vi "Start Stop Integration.vi"(0 "VISA resource name":refnum<visa-resource-name>, 5 "Start/Stop (F: Stop)":bool, 11 "error in (no error)":errorcluster) -> (4 "VISA resource name out":refnum<visa-resource-name>, 15 "error out":errorcluster)   [LabVIEW 2011, in "Yokogawa WT200 Series.lvlib"]
doc: "This VI sends the Integrate start/stop command to the WT200 Series."
uses:
  G:/Engineering/Retail/LabV/instr.lib/Yokogawa WT200 Series/Yokogawa WT200 Series.lvlib
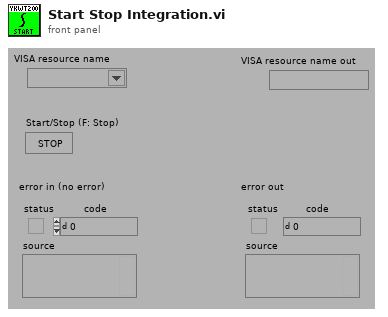
[diagram p1: front panel]
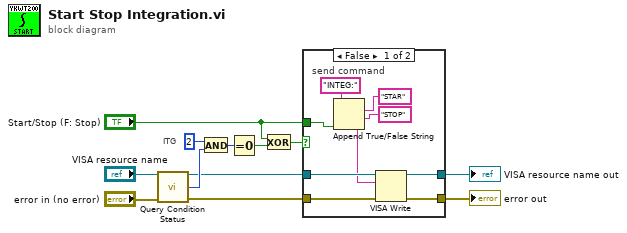
[diagram p0: block diagram]
diagram:
  # "ITG"
  n1 = call <instrlib>:"Query Condition Status.vi"("VISA resource name"="VISA resource name", "error in (no error)"="error in (no error)") -> ("VISA resource name out"=w2:refnum<visa-resource-name>, "Condition"=w3:u16, "error out"=w7:errorcluster)  [unwired: 11 in]
  n2 = And(x=u16 2, y=w3) -> (x .and. y?=w8:u16)
  n3 = Equal To 0?(x=w8) -> (x = 0?=w9:bool)
  n4 = Exclusive Or(1:w9, 2:"Start/Stop (F: Stop)") -> (0:w10:bool)
  n5 = case shown="False" w10 {
    tunnel: w7 -> [w17 w23]
    tunnel: [w16 w23] -> w12
    tunnel: "Start/Stop (F: Stop)" -> [w18 _]
    tunnel: w2 -> [w15 w22]
    tunnel: [w14 w22] -> w1
    frame False {
      # "send command"
      n6 = Append True/False String(1:w18, 2:"STOP", 3:"STAR", 4:"INTEG:") -> (0:w13:string)
      n7 = VISA Write(VISA resource name=w15, write buffer=w13, error in (no error)=w17) -> (VISA resource name out=w14:refnum<visa-resource-name>, error out=w16:errorcluster)  [unwired: 1 out]
    }
    frame True {
      # "no change"
    }
  }
  "error out" <- w12
  "VISA resource name out" <- w1
